vi "Populate Menu from Graph Items.vi"(5 "Parent Tag (None)":string, 7 "Menu":refnum<k9>, 10 "Selected Item (None)":i32=-1, 11 "Items":T1[](array[typedef])) -> ()   [LabVIEW 2020, in "TypeGraph.lvlib"]
uses:
  TypeGraph.lvlib
  Type Reflection Item.ctl
  <vilib>/Utility/Data Type/NI_Data Type.lvlib
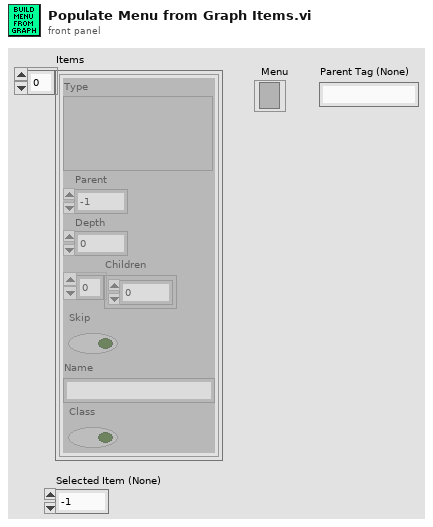
[diagram p1: front panel]
types:
  T1 = typedef "TypeGraph.lvlib/Type Reflection Item.ctl" = cluster{"Type":variant, "Parent":i32, "Depth":i32, "Children":i32[], "Skip":bool, "Name":string, "Class":bool}
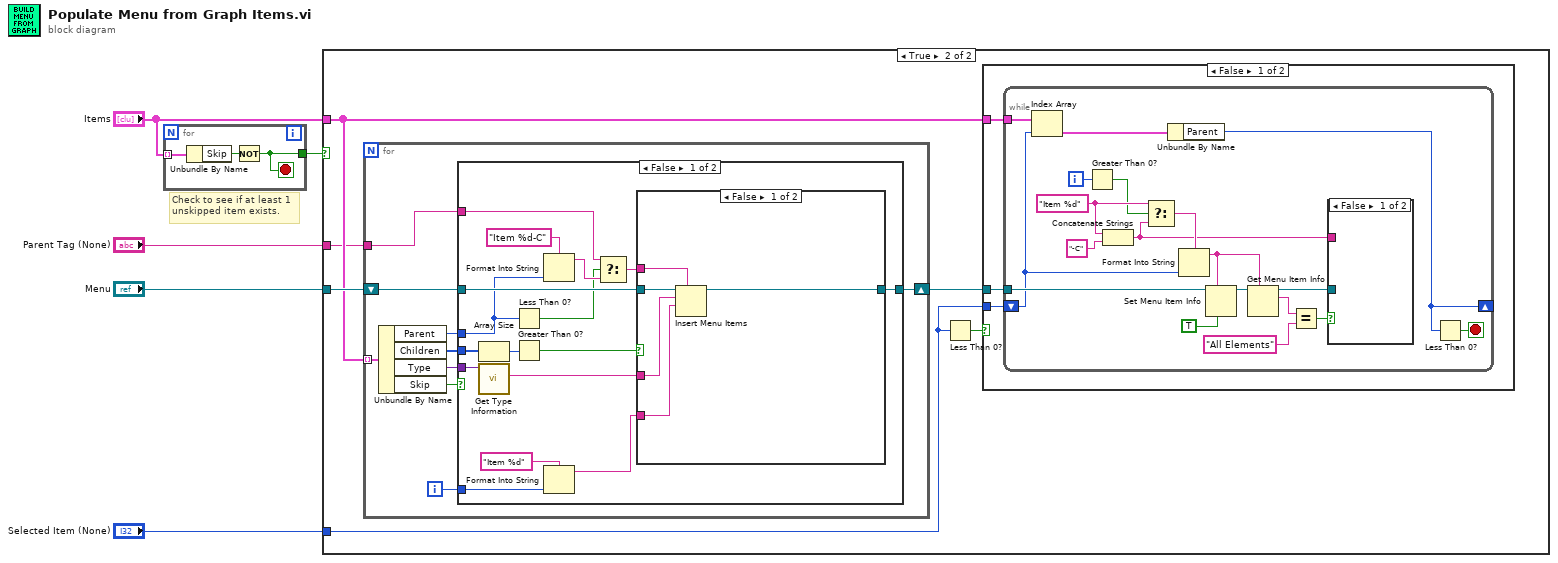
[diagram p0: block diagram]
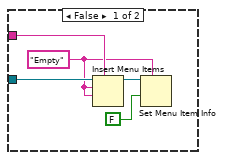
[diagram p2: hidden frame]
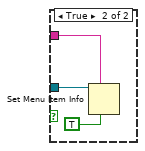
[diagram p3: hidden frame]
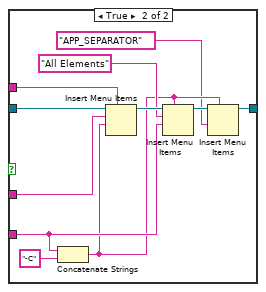
[diagram p5: hidden frame]
diagram:
  # "Check to see if at least 1 unskipped item exists."
  n1 = for {
    tunnel: "Items" -> [w8] mode=indexing
    tunnel: [w6] -> w2
    stop <- w6 stop-if-true
    n2 = Unbundle By Name(w8) -> ("Skip"=w7:bool)
    n3 = Not(x=w7) -> (.not. x?=w6:bool)
  }
  n4 = case shown="True" w2 {
    tunnel: "Items" -> [_ w17]
    tunnel: "Menu" -> [w13 w19]
    tunnel: "Selected Item (None)" -> [_ w15]
    tunnel: "Parent Tag (None)" -> [w10 w16]
    frame False {
      w9 = "Empty"
      n5 = Insert Menu Items(5:w10, 7:w9, 8:w9, 9:w13) -> (3:w12:refnum<k9>)  [unwired: 2 in, 2 out]
      n6 = Set Menu Item Info(7:w9, 9:FALSE ("enabled"), 11:w12) -> ()  [unwired: 4 in, 2 out]
    }
    frame True {
      n7 = for {
        tunnel: w17 -> [w53] mode=indexing
        shift-right: [w46] -> w18
        shift-left: w19 -> [w49]
        tunnel: w16 -> [w45]
        i -> [w48]
        n8 = Unbundle By Name(w53) -> ("Parent"=w47:i32, "Children"=w50:i32[], "Type"=w51:variant, "Skip"=w52:bool)
        n9 = case shown="False" w52 {
          tunnel: w51 -> [w56 _]
          tunnel: w50 -> [w69 _]
          tunnel: w49 -> [w65 w86]
          tunnel: w48 -> [w67 _]
          tunnel: w47 -> [w57 _]
          tunnel: [w62 w86] -> w46
          tunnel: w45 -> [w54 _]
          frame False {
            n10 = Array Size(array=w69) -> (size(s)=w68:i32)
            n11 = call <vilib>:"Get Type Information.vi"("variant"=w56) -> ("name"=w55:string)  [unwired: 6 in, 4 out]
            n12 = Less Than 0?(x=w57) -> (x < 0?=w59:bool)
            n13 = Greater Than 0?(x=w68) -> (x > 0?=w66:bool)
            n14 = Format Into String(format string="Item %d-C", w57) -> (resulting string=w61:string)  [unwired: 2 in, 1 out]
            n15 = Format Into String(format string="Item %d", w67) -> (resulting string=w64:string)  [unwired: 2 in, 1 out]
            n16 = Select(t=w54, s=w59, f=w61) -> (s? t:f=w60:string)
            n17 = case shown="False" w66 {
              tunnel: w65 -> [w74 w84]
              tunnel: w64 -> [w72 w80]
              tunnel: w55 -> [w71 w83]
              tunnel: w60 -> [w73 w75]
              tunnel: [w70 w76] -> w62
              frame False {
                n18 = Insert Menu Items(5:w73, 7:w72, 8:w71, 9:w74) -> (3:w70:refnum<k9>)  [unwired: 2 in, 2 out]
              }
              frame True {
                n19 = Concatenate Strings(w80, "-C" ("string")) -> (w78:string)
                n20 = Insert Menu Items(5:w75, 7:w78, 8:w83, 9:w84) -> (3:w82:refnum<k9>)  [unwired: 2 in, 2 out]
                n21 = Insert Menu Items(5:w78, 7:w80, 8:"All Elements", 9:w82) -> (3:w79:refnum<k9>)  [unwired: 2 in, 2 out]
                n22 = Insert Menu Items(5:w78, 7:"APP_SEPARATOR", 9:w79) -> (3:w76:refnum<k9>)  [unwired: 3 in, 2 out]
              }
            }
          }
          frame True {
          }
        }
      }
      n23 = Less Than 0?(x=w15) -> (x < 0?=w14:bool)
      n24 = case shown="False" w14 {
        tunnel: w18 -> [w22 _]
        tunnel: w15 -> [w21 _]
        tunnel: w17 -> [w20 _]
        frame False {
          n25 = while {
            tunnel: w22 -> [w40]
            shift-right: [w37] -> _
            shift-left: w21 -> [w36]
            tunnel: w20 -> [w39]
            i -> [w29]
            stop <- w41 stop-if-true
            w26 = "Item %d"
            n26 = Index Array(array=w39, index=w36) -> (element=w38:T1)
            n27 = Greater Than 0?(x=w29) -> (x > 0?=w24:bool)
            n28 = Concatenate Strings(w26, "-C" ("string")) -> (w23:string)
            n29 = Select(t=w26, s=w24, f=w23) -> (s? t:f=w25:string)
            n30 = Unbundle By Name(w38) -> ("Parent"=w37:i32)
            n31 = Format Into String(format string=w25, w36) -> (resulting string=w30:string)  [unwired: 2 in, 1 out]
            n32 = Set Menu Item Info(6:TRUE ("checked"), 7:w30, 11:w40) -> (3:w34:refnum<k9>)  [unwired: 4 in, 1 out]
            n33 = Get Menu Item Info(7:w30, 11:w34) -> (2:w33:string, 3:w31:refnum<k9>)  [unwired: 1 in, 5 out]
            n34 = Equal?(x=w33, y="All Elements") -> (x = y?=w28:bool)
            n35 = case shown="False" w28 {
              tunnel: w31 -> [_ w44]
              tunnel: w23 -> [_ w42]
              frame False {
              }
              frame True {
                n36 = Set Menu Item Info(6:TRUE ("checked"), 7:w42, 11:w44) -> ()  [unwired: 4 in, 2 out]
              }
            }
            n37 = Less Than 0?(x=w37) -> (x < 0?=w41:bool)
          }
        }
        frame True {
        }
      }
    }
  }
